vi "Load Classes.vi"(8 "error in (no error)":errorcluster, 10 "class paths":path[](array[path]), 11 "Component Loader in":refnum<class "Component Loader.lvclass">) -> (0 "error out":errorcluster, 2 "objects":refnum<class>[](array[class]), 3 "Component Loader out":refnum<class "Component Loader.lvclass">)   [LabVIEW 2019, in "DSF Core.lvlib" / "Component Loader.lvclass"]
uses:
  Component Loader.lvclass
  Errors.vi
  Class Not Found.vi
  New Component Loader Error.vi
  <vilib>/NI/Memory Manager/VIs/Write String to Source.vi
  <vilib>/NI/Memory Manager/VIs/New Error Cluster.vi
  <vilib>/NI/Memory Manager/VIs/New Error Cluster (512B).vi
  Component Loader Error Info.vi
  <vilib>/NI/Memory Manager/VIs/Set Error Code.vi
  <vilib>/NI/Memory Manager/VIs/Set Error Status.vi
  <vilib>/NI/Memory Manager/VIs/Set Error Source.vi
  VIs/Constants/Constants.vi
  VIs/Constants/Engine Library Name.vi
  Base Error Offset.vi
  VIs/Constants/Base Error Code.vi
  <vilib>/Utility/libraryn.llb/Check if File or Folder Exists.vi
  <vilib>/Utility/LVClass/Get LV Class Default Value.vi
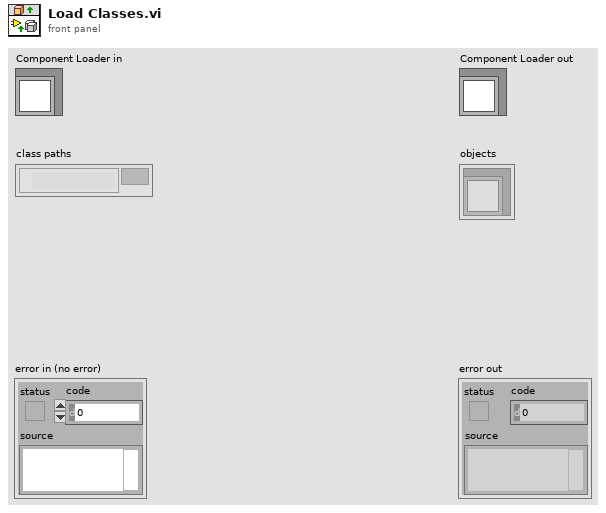
[diagram p1: front panel]
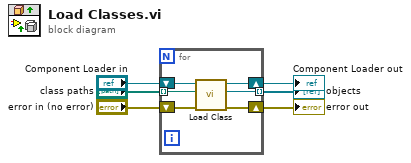
[diagram p0: block diagram]
diagram:
  n1 = for {
    tunnel: [w12] -> w5 mode=indexing
    shift-right: [w11] -> w3
    shift-left: "Component Loader in" -> [w10]
    tunnel: "class paths" -> [w9] mode=indexing
    shift-right: [w8] -> w2
    shift-left: "error in (no error)" -> [w7]
    n2 = call "Load Class.vi"("error in (no error)"=w7, "class path"=w9, "Component Loader in"=w10) -> ("error out"=w8:errorcluster, "object"=w12:refnum<class>, "Component Loader out"=w11:refnum<class "Component Loader.lvclass">)  [unwired: 6 in]
  }
  "error out" <- w2
  "Component Loader out" <- w3
  "objects" <- w5
